vi "Status.vi"(8 "error in (no error)":errorcluster, 11 "SS P100 Settings In":T1) -> (0 "error out":errorcluster, 1 "Connection Error":bool, 2 "Running":bool, 3 "SS P100 Settings Out":T1, 4 "Power":i32, 5 "Amplitude":i32)   [LabVIEW 2018, in "Sonic Systems P100.lvlib"]
uses:
  Sonic Systems P100.lvlib
  Sonic Systems P100 Settings.ctl
  <vilib>/regexp/Match Regular Expression.xnode
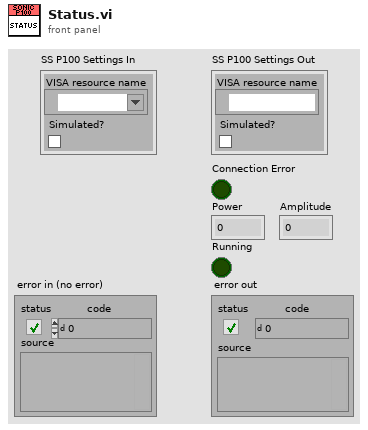
[diagram p1: front panel]
types:
  T1 = typedef "Sonic Systems P100.lvlib/Sonic Systems P100 Settings.ctl" = cluster{"VISA resource name":refnum<visa-resource-name>, "Simulated?":bool}
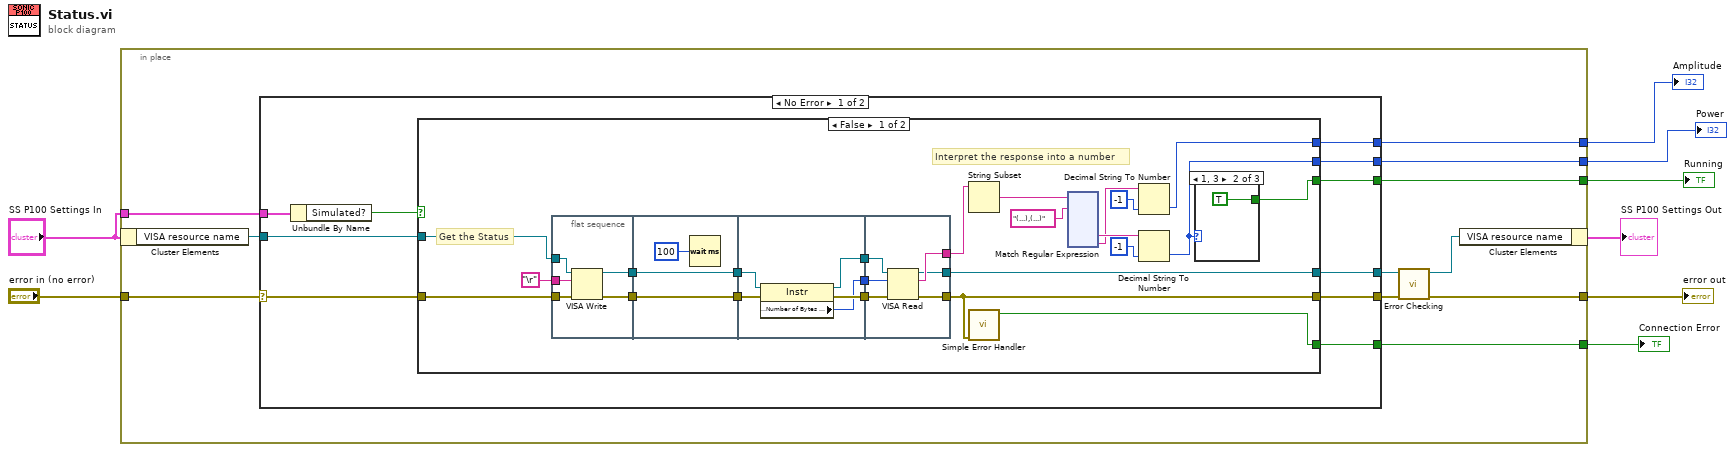
[diagram p0: block diagram]
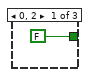
[diagram p2: hidden frame]
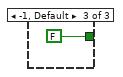
[diagram p3: hidden frame]
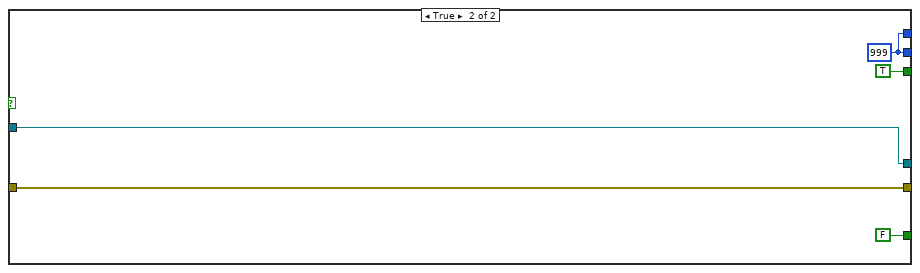
[diagram p4: hidden frame]
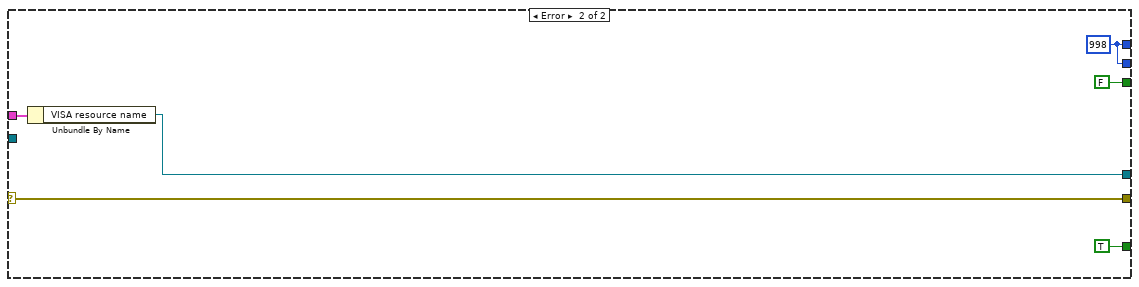
[diagram p5: hidden frame]
diagram:
  n1 = in-place {
    in-place-border: "error in (no error)" -> [w19]
    in-place-border: [w16] -> w7
    in-place-border: "SS P100 Settings In" -> [w15]
    in-place-border: [w12] -> w4
    in-place-border: [w10] -> w3
    in-place-border: [w11] -> w2
    in-place-border: [w9] -> w1
    n2 = in-place-cluster #1("SS P100 Settings In") -> ("VISA resource name"=w14:refnum<visa-resource-name>)
    n3 = case shown="No Error" w19 {
      selector: w19 -> [w29 w202]
      tunnel: w15 -> [w27 w201]
      tunnel: [w28 w202] -> w17
      tunnel: [w26 w200] -> w18
      tunnel: [w24 TRUE] -> w12
      tunnel: [w23 FALSE] -> w11
      tunnel: w14 -> [w22 _]
      tunnel: [w21 w197] -> w10
      tunnel: [w20 w197] -> w9
      frame No Error {
        n4 = Unbundle By Name(w27) -> ("Simulated?"=w25:bool)
        n5 = case shown="False" w25 {
          tunnel: w29 -> [w42 w196]
          tunnel: [w34 w196] -> w28
          tunnel: [w44 w195] -> w26
          tunnel: w22 -> [w43 w195]
          tunnel: [w33 FALSE] -> w24
          tunnel: [w41 TRUE] -> w23
          tunnel: [w38 w192] -> w21
          tunnel: [w30 w192] -> w20
          frame False {
            # "Interpret the response into a number"
            # "Get the Status"
            n6 = flat-sequence {
              tunnel: [w177] -> w52
              tunnel: [w176] -> w51
              tunnel: w43 -> [w175]
              tunnel: w42 -> [w174]
              tunnel: "\r" -> [w173]
              tunnel: w52 -> [w179]
              tunnel: w51 -> [w178]
              tunnel: [w179] -> w46
              tunnel: [w178] -> w45
              tunnel: [w183] -> w49
              tunnel: [w182] -> w48
              tunnel: [w181] -> w47
              tunnel: w46 -> [w185]
              tunnel: w45 -> [w184]
              tunnel: [w191] -> w34
              tunnel: [w190] -> w50
              tunnel: [w189] -> w44
              tunnel: w49 -> [w188]
              tunnel: w48 -> [w187]
              tunnel: w47 -> [w186]
              frame #0 {
                n7 = VISA Write(VISA resource name=w175, write buffer=w173, error in (no error)=w174) -> (VISA resource name out=w177:refnum<visa-resource-name>, error out=w176:errorcluster)  [unwired: 1 out]
              }
              frame #1 {
                n8 = Wait (ms)(milliseconds to wait=u32 100) -> ()  [unwired: 1 out]
              }
              frame #2 {
                n9 = property class="Instr"(reference=w185, error in=w184) -> (reference out=w183:refnum<visa-resource-name>, error out=w182:errorcluster, "Serial Settings:Number of Bytes at Serial Port"=w181:u32)
              }
              frame #3 {
                n10 = VISA Read(VISA resource name=w188, byte count=w186, error in (no error)=w187) -> (VISA resource name out=w189:refnum<visa-resource-name>, read buffer=w190:string, error out=w191:errorcluster)  [unwired: 1 out]
              }
            }
            n11 = String Subset(string=w50) -> (substring=w37:string)  [unwired: 2 in]
            n12 = call <vilib>:"Simple Error Handler.vi"("error in (no error)"=w34) -> ("error?"=w33:bool)  [unwired: 4 in, 4 out]
            n13 = xnode "Match Regular Expression"("input string"=w37, "regular expression"="(...),(...)") -> ("submatch 1"=w35:string, "submatch 2"=w31:string)  [unwired: 4 in, 5 out]
            n14 = Decimal String To Number(string=w31, default (0L)=-1 ("default (0 I32)")) -> (number=w30:i32)  [unwired: 1 in, 1 out]
            n15 = Decimal String To Number(string=w35, default (0L)=-1 ("default (0 I32)")) -> (number=w38:i32)  [unwired: 1 in, 1 out]
            n16 = case shown="1, 3" w38 {
              tunnel: [FALSE TRUE FALSE] -> w41
              frame 0, 2 {
              }
              frame 1, 3 {
              }
              frame -1, Default {
              }
            }
          }
          frame True {
            w192 = 999
          }
        }
      }
      frame Error {
        w197 = 998
        n17 = Unbundle By Name(w201) -> ("VISA resource name"=w200:refnum<visa-resource-name>)
      }
    }
    n18 = call "Error Checking.vi"("error in (no error)"=w17, "VISA resource name"=w18) -> ("error out"=w16:errorcluster, "VISA resource name"=w13:refnum<visa-resource-name>)  [unwired: 7 in, 1 out]
    n19 = in-place-cluster #1("VISA resource name"=w13) -> (→"SS P100 Settings Out":T1)
  }
  "error out" <- w7
  "Connection Error" <- w4
  "Power" <- w3
  "Running" <- w2
  "Amplitude" <- w1
